vi "SW_Prepare_TTL_activation_sequence.vi"(8 "Error In":errorcluster, 9 "Settings cluster (local)":T1 {"Calibration parameters"."True frame time, s" format="%.10g"; "Calibration parameters"."Disp. calibration info"."Speed, µl per ms" format="%.3g"; "Calibration parameters"."True FPS" format="%.10g"; "Calibration parameters"."Timing calibration sw/hw" format="%.10g"; "Conditions presets array"."Specifier(s)"."Validity criteria(s)"."Validity value" min=0.0 step=0.1 format="%.2g"; "Conditions presets array"."Specifier(s)"."Value" step=1.0 format="%#.2g"; "Recording and saving"."Data post-processing"."Order" min=3 max=11 step=2; "Recording and saving"."Data post-processing"."Length" min=5 max=301 step=2; "Geometry"."Cage diameter, mm" scale=0.0..340.0}, 11 "Rules (conditions) to activate":bool[](array[boolean])=[FALSE, FALSE, FALSE, FALSE]) -> (0 "Error Out":errorcluster, 3 "TTL out sequence":cluster{"Numeric":dbl, "String":string}[](array[cluster]))   [LabVIEW 2018, in "Tracker.lvlib"]
uses:
  Tracker.lvlib
  Controls/CTL_Settings_cluster.ctl
  Controls/CTL_Histogram_parameters.ctl
  Controls/CTL_Filter_selector.ctl
  Controls/CTL_Acquisition_speed_selector.ctl
  Controls/CTL_Segmented_plot_parameters.ctl
  Controls/CTL_IO_params_cluster.ctl
  Controls/CTL_Conditions_Array.ctl
  Controls/CTL_Conditions_Cluster.ctl
  Controls/CTL_Condition_type.ctl
  Controls/CTL_Comparison_type.ctl
  Controls/CTL_Validity_check_criteria.ctl
  Controls/CTL_Response_info.ctl
  Controls/CTL_Condition_response_type.ctl
  Controls/CTL_Reponse_port_info.ctl
  Controls/CTL_Calibration_parameters.ctl
  Controls/CTL_Dispenser_calibration_info.ctl
  <userlib>/_OpenG.lib/array/array.llb/Sort 1D Array (DBL)__ogtk.vi
  <userlib>/_OpenG.lib/array/array.llb/Reorder 1D Array2 (U8)__ogtk.vi
  <userlib>/_OpenG.lib/array/array.llb/Remove Duplicates from 1D Array (U8)__ogtk.vi
  <userlib>/_OpenG.lib/array/array.llb/Search 1D Array (DBL)__ogtk.vi
  <userlib>/_OpenG.lib/array/array.llb/Delete Elements from 1D Array (U8)__ogtk.vi
  <userlib>/_OpenG.lib/array/array.llb/Delete Elements from 1D Array (DBL)__ogtk.vi
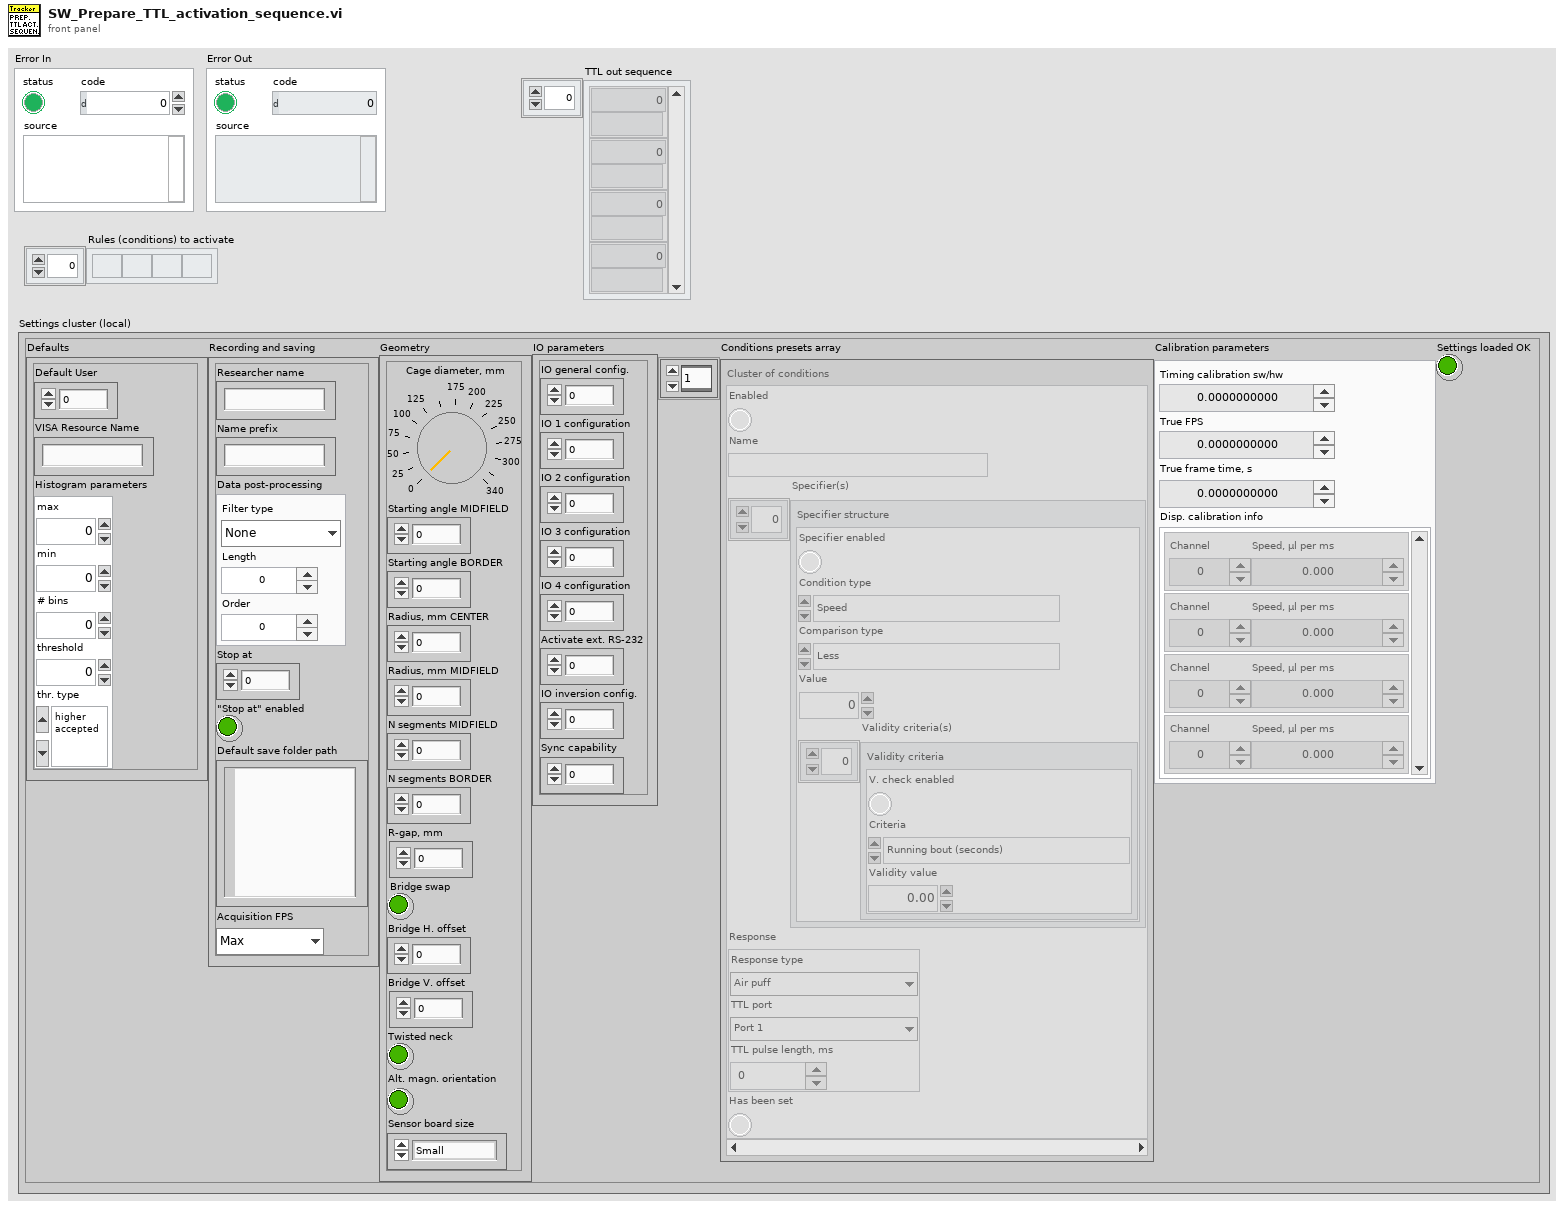
[diagram p1: front panel]
types:
  T1 = typedef "Tracker.lvlib/CTL_Settings_cluster.ctl" = cluster{"Defaults":cluster{"Default User":dbl, "VISA Resource Name ":string, "Histogram parameters":T2}, "Recording and saving":cluster{"Researcher name":string, "Name prefix":string, "Data post-processing":T3, "Stop at":dbl, "\"Stop at\" enabled":bool, "Default save folder path":path, "Acquisition FPS":T4}, "Geometry":T5, "IO parameters":T6, "Conditions presets array":T7, "Calibration parameters":T15, "Settings loaded OK":bool}
  T2 = typedef "Tracker.lvlib/CTL_Histogram_parameters.ctl" = cluster{"max":dbl, "min":dbl, "# bins":i32, "threshold":dbl, "thr. type":enum16{"higher accepted", "lower accepted"}}
  T3 = typedef "Tracker.lvlib/CTL_Filter_selector.ctl" = cluster{"Filter type":enum16{"None", "Savitzky-Golay"}, "Length":i32, "Order":i32}
  T4 = typedef "Tracker.lvlib/CTL_Acquisition_speed_selector.ctl" = enum16{"Max", "Optimal", "Eco"}
  T5 = typedef "Tracker.lvlib/CTL_Segmented_plot_parameters.ctl" = cluster{"Cage diameter, mm":u16, "Starting angle MIDFIELD":i16, "Starting angle BORDER":i16, "Radius, mm CENTER":u16, "Radius, mm MIDFIELD":u16, "N segments MIDFIELD":u8, "N segments BORDER":u8, "R-gap, mm":sgl, "Bridge swap":bool, "Bridge H. offset":sgl, "Bridge V. offset":sgl, "Twisted neck":bool, "Alt. magn. orientation":bool, "Sensor board size":enum16{"Small", "Large"}}
  T6 = typedef "Tracker.lvlib/CTL_IO_params_cluster.ctl" = cluster{"IO general config.":u16, "IO 1 configuration":u16, "IO 2 configuration":u16, "IO 3 configuration":u16, "IO 4 configuration":u16, "Activate ext. RS-232":u16, "IO inversion config.":u16, "Sync capability":u8}
  T7 = typedef "Tracker.lvlib/CTL_Conditions_Array.ctl" = T8[]
  T8 = typedef "Tracker.lvlib/CTL_Conditions_Cluster.ctl" = cluster{"Enabled":bool, "Name":string, "Specifier(s)":cluster{"Specifier enabled":bool, "Condition type":T9, "Comparison type":T10, "Value":dbl, "Validity criteria(s)":cluster{"V. check enabled":bool, "Criteria":T11, "Validity value":dbl}[]}[], "Response":T12, "Has been set":bool}
  T9 = typedef "Tracker.lvlib/CTL_Condition_type.ctl" = enum16{"Speed", "Zone", "Angle to wall"}
  T10 = typedef "Tracker.lvlib/CTL_Comparison_type.ctl" = enum16{"Less", "Less or Equal", "Equal", "Greater or Equal", "Greater", "Not Equal"}
  T11 = typedef "Tracker.lvlib/CTL_Validity_check_criteria.ctl" = enum16{"Running bout (seconds)", "Running bout (meters)"}
  T12 = typedef "Tracker.lvlib/CTL_Response_info.ctl" = cluster{"Response type":T13, "TTL port":T14, "TTL pulse length, ms":dbl}
  T13 = typedef "Tracker.lvlib/CTL_Condition_response_type.ctl" = enum16{"None", "Air puff", "Liquid reward"}
  T14 = typedef "Tracker.lvlib/CTL_Reponse_port_info.ctl" = enum16{"Port 1", "Port 2", "Port 3", "Port 4"}
  T15 = typedef "Tracker.lvlib/CTL_Calibration_parameters.ctl" = cluster{"Timing calibration sw/hw":dbl, "True FPS":dbl, "True frame time, s":dbl, "Disp. calibration info":T16}
  T16 = typedef "Tracker.lvlib/CTL_Dispenser_calibration_info.ctl" = cluster{"Channel":u8, "Speed, µl per ms":dbl}[]
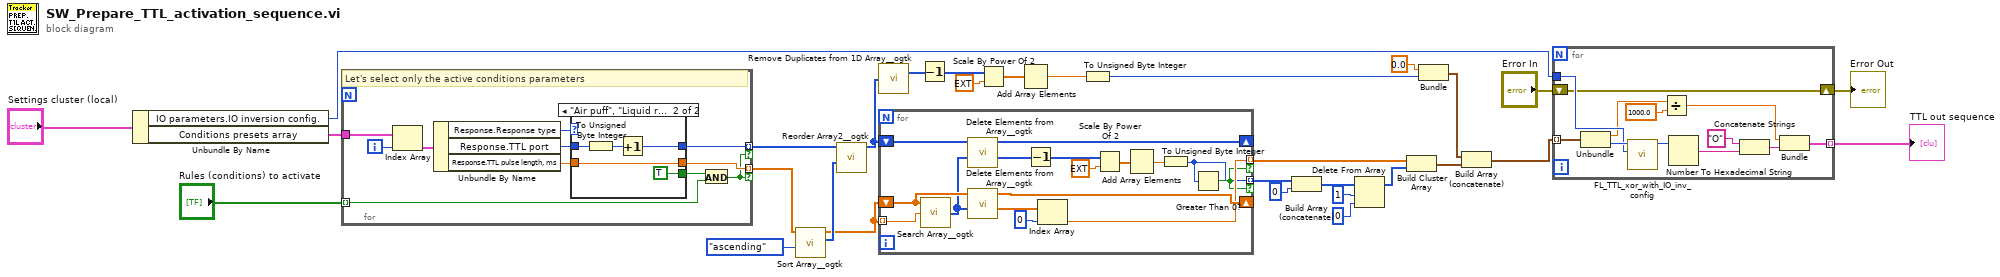
[diagram p0: block diagram]
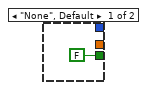
[diagram p2: hidden frame]
diagram:
  n1 = Unbundle By Name("Settings cluster (local)") -> ("IO parameters.IO inversion config."=w17:u16, "Conditions presets array"=w30:T7)
  n2 = for {
    tunnel: "Rules (conditions) to activate" -> [w36] mode=indexing
    tunnel: w30 -> [w41]
    tunnel: [w33] -> w11 mode=indexing if=w31
    tunnel: [w32] -> w9 mode=indexing if=w31
    i -> [w34]
    # "Let's select only the active conditions parameters"
    n3 = Index Array(array=w41, index=w34) -> (element=w40:T8)
    n4 = Unbundle By Name(w40) -> ("Response.Response type"=w39:T13, "Response.TTL port"=w38:T14, "Response.TTL pulse length, ms"=w37:dbl)
    n5 = case shown="\"Air puff\", \"Liquid reward\"" w39 {
      tunnel: w38 -> [_ w44]
      tunnel: w37 -> [_ w46]
      tunnel: [FALSE TRUE] -> w35
      tunnel: [_ w46] -> w33
      tunnel: [_ w43] -> w32
      frame "None", Default {
      }
      frame "Air puff", "Liquid reward" {
        n6 = To Unsigned Byte Integer(number=w44) -> (unsigned 8bit integer=w45:u8)
        n7 = Increment(x=w45) -> (x+1=w43:u8)
      }
    }
    n8 = And(x=w35, y=w36) -> (x .and. y?=w31:bool)
  }
  n9 = call-poly <userlib>:"Sort Array__ogtk.vi"("Order"=enum16{"ascending", "descending"}."ascending", "Array in"=w11) -> ("Sorted Pointers"=w8:i32[], "Sorted Array out"=w7:dbl[])  [unwired: 8 in]
  n10 = call-poly <userlib>:"Reorder Array2__ogtk.vi"("indices"=w8, "array"=w9) -> ("reordered array"=w6:u8[])  [unwired: 9 in]
  n11 = call-poly <userlib>:"Remove Duplicates from 1D Array__ogtk.vi"("Input Array"=w6) -> ("Output Array"=w27:u8[])  [unwired: 1 out]
  n12 = for {
    tunnel: w7 -> [w63] mode=indexing
    shift-right: [w61] -> _
    shift-left: w7 -> [w62]
    shift-right: [w57] -> _
    shift-left: w6 -> [w59]
    tunnel: [w55] -> w20 mode=indexing if=w53
    tunnel: [w48] -> w25 mode=indexing if=w53
    n13 = call-poly <userlib>:"Search Array__ogtk.vi"("Array"=w62, "Element Data"=w63) -> ("Indices of Elements"=w58:i32[])  [unwired: 7 in]
    n14 = call-poly <userlib>:"Delete Elements from Array__ogtk.vi"("indices"=w58, "array"=w59) -> ("deleted elements"=w50:u8[], "array w/ subset deleted"=w57:u8[])  [unwired: 8 in]
    n15 = call-poly <userlib>:"Delete Elements from Array__ogtk.vi"("indices"=w58, "array"=w62) -> ("deleted elements"=w60:dbl[], "array w/ subset deleted"=w61:dbl[])  [unwired: 8 in]
    n16 = Decrement(x=w50) -> (x-1=w51:u8[])
    n17 = Index Array(array=w60, index=0) -> (element=w55:dbl)
    n18 = Scale By Power Of 2(n=w51, x=ext 1.0) -> (x*2^n=w49:ext[])
    n19 = Add Array Elements(numeric array=w49) -> (sum=w54:ext)
    n20 = To Unsigned Byte Integer(number=w54) -> (unsigned 8bit integer=w48:u8)
    n21 = Greater Than 0?(x=w48) -> (x > 0?=w53:bool)
  }
  n22 = Decrement(x=w27) -> (x-1=w2:u8[])
  n23 = Scale By Power Of 2(n=w2, x=ext 1.0) -> (x*2^n=w5:ext[])
  n24 = Add Array Elements(numeric array=w5) -> (sum=w12:ext)
  n25 = To Unsigned Byte Integer(number=w12) -> (unsigned 8bit integer=w3:u8)
  n26 = Build Array (concatenate)(w25, u8 0) -> (w23:u8[])
  n27 = Delete From Array(array=w23, length=1, index=0) -> (array with subset deleted=w1:u8[])  [unwired: 1 out]
  n28 = Build Cluster Array(w20, w1) -> (w19:cluster{dbl, u8}[])
  n29 = Bundle(0.0, w3) -> (w14:cluster{dbl, u8})  [unwired: 1 in]
  n30 = Build Array (concatenate)(w14, w19) -> (w15:cluster{dbl, u8}[])
  n31 = for {
    shift-right: [w69] -> w18
    shift-left: "Error In" -> [w69]
    tunnel: w15 -> [w75] mode=indexing
    tunnel: w17 -> [w71]
    tunnel: [w64] -> w13 mode=indexing
    n32 = Unbundle(w75) -> (w67:dbl, w72:u8)
    n33 = call "FL_TTL_xor_with_IO_inv_config.vi"("IO inversion config."=w71, "TTL port(s) config to fire"=w72) -> ("ON config."=w70:u32)  [unwired: 8 in, 1 out]
    n34 = Divide(x=w67, y=1000.0) -> (x/y=w66:dbl)
    n35 = Number To Hexadecimal String(2:w70) -> (0:w74:string)  [unwired: 1 in]
    n36 = Concatenate Strings("O" ("string"), w74) -> (w68:string)
    n37 = Bundle(w66, w68) -> (w64:cluster{dbl, string})  [unwired: 1 in]
  }
  "Error Out" <- w18
  "TTL out sequence" <- w13
